vi "ecu_module.vi"(8 "error in (no error)":errorcluster, 10 "ecuData":refnum<user-event>, 11 "queue in":T1) -> (0 "error out":errorcluster)   [LabVIEW 2019]
uses:
  core_dataRef.ctl
  core_dataCluster.ctl
  gui/ecu_dataCluster.ctl
  instrument/Instrument.lvclass
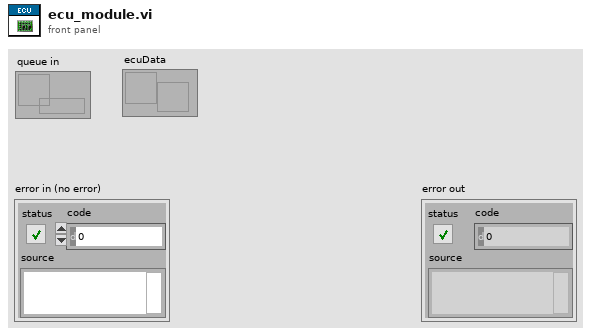
[diagram p1: front panel]
types:
  T1 = typedef "core_dataRef.ctl" = refnum<queue>
  T2 = typedef "ecu_dataCluster.ctl" = cluster{"MCU_MotCtrlrSts":dbl, "MCU_MotTq":dbl, "MCU_MotBusU":dbl, "MCU_MotSpd":dbl, "MCU_MotBodyT":dbl, "MCU_MotBody_T":dbl, "MCU_MotCtrlrT":dbl, "MCU 状态":bool, "ErrMsg":i64}
  T3 = typedef "core_dataCluster.ctl" = cluster{"cmd":string, "data":variant}
  T4 = typedef "Instrument.lvclass/DUT_Status.ctl" = cluster{"MCU_MotCtrlrSts":sgl, "MCU_MotTq":sgl, "MCU_MotBusU":sgl, "MCU_MotSpd":sgl}
  T5 = typedef "Instrument.lvclass/DUT_Temp.ctl" = cluster{"0x149_MCU_MotBodyT":sgl, "0x304_MCU_MotBodyT":sgl, "0x304_MCU_MotCtrlrT":sgl}
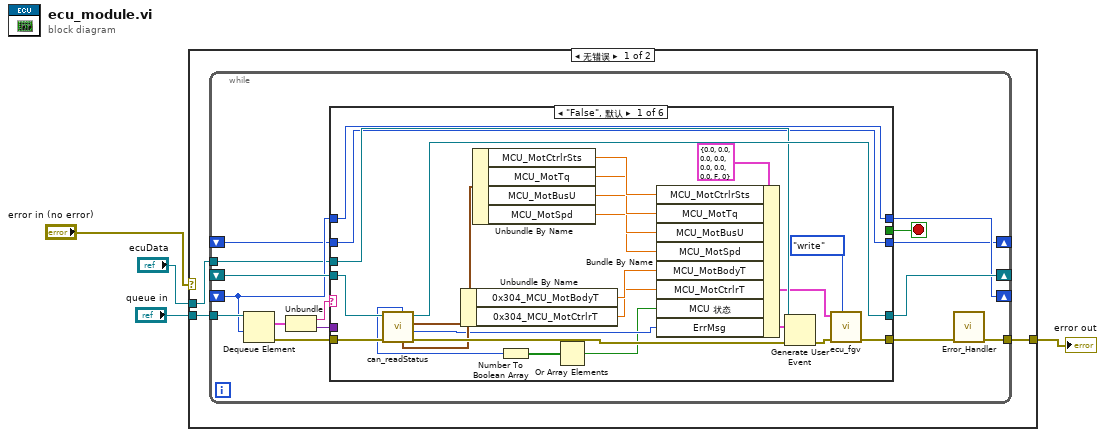
[diagram p0: block diagram]
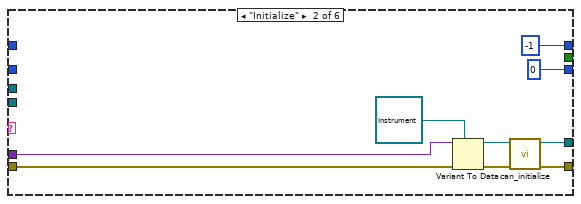
[diagram p2: hidden frame]
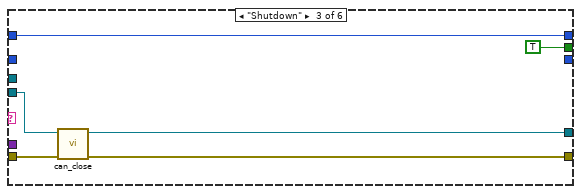
[diagram p3: hidden frame]
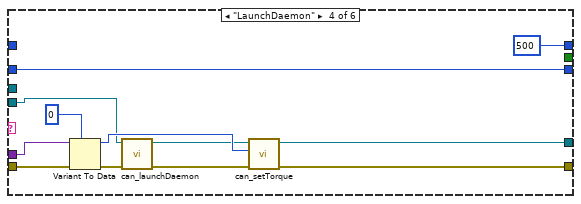
[diagram p4: hidden frame]
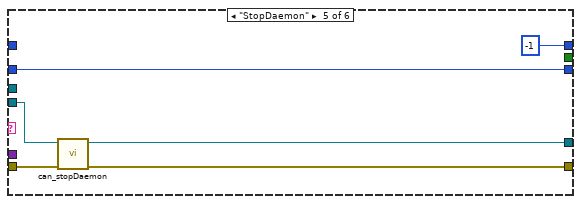
[diagram p5: hidden frame]
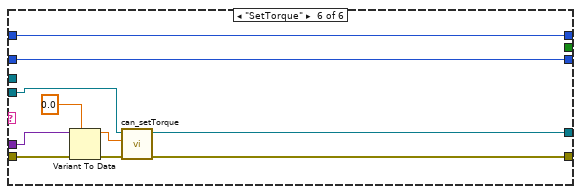
[diagram p6: hidden frame]
diagram:
  n1 = case shown="无错误" "error in (no error)" {
    selector: "error in (no error)" -> [_ w90]
    tunnel: "queue in" -> [w7 _]
    tunnel: [w6 w90] -> w3
    tunnel: "ecuData" -> [w5 _]
    frame No Error {
      n2 = while {
        tunnel: w7 -> [w22]
        shift-right: [w17] -> _
        shift-left: _ -> [w16]
        tunnel: [w14] -> w6
        shift-right: [w13] -> _
        shift-left: _ -> [w12]
        tunnel: w5 -> [w11]
        shift-right: [w10] -> _
        shift-left: _ -> [w9]
        stop <- w15 stop-if-true
        n3 = Dequeue Element(queue=w22, timeout in ms (-1)=w12) -> (element=w21:T3, error out=w19:errorcluster)  [unwired: 1 in, 2 out]
        n4 = Unbundle(w21) -> ("cmd"=w20:string, "data"=w18:variant)
        n5 = case shown="\"False\", 默认" w20 {
          tunnel: w19 -> [w43 w55 w57 w72 w78 w89]
          tunnel: w18 -> [_ w54 _ w71 _ w88]
          tunnel: [w44 w50 w61 w68 w77 w83] -> w17
          tunnel: w16 -> [w45 _ w58 w66 w79 w86]
          tunnel: [w39 w49 w60 w69 w76 w82] -> w8
          tunnel: [_ _ TRUE _ _ _] -> w15
          tunnel: [w46 -1 ("timeout in ms (-1)") w56 500 ("timeout in ms (-1)") -1 ("timeout in ms (-1)") w81] -> w13
          tunnel: w12 -> [w46 _ w56 _ _ w81]
          tunnel: w11 -> [w42 _ _ _ _ _]
          tunnel: [w37 u8 0 ("Control Mode") _ w64 w74 w80] -> w10
          tunnel: w9 -> [w37 _ _ w64 w74 w80]
          frame "False", Default {
            n6 = call "can_readStatus.vi"("error in (no error)"=w43, "Instrument in"=w45) -> ("error out"=w41:errorcluster, "FaultCode"=w26:u8, "Cluster"=w36:T4, "Instrument out"=w44:refnum<class "Instrument.lvclass">, "DUT_Temp"=w35:T5, "ReFltLvl"=w24:u8)  [unwired: 4 in]
            n7 = Unbundle By Name(w35) -> ("0x304_MCU_MotBodyT"=w28:sgl, "0x304_MCU_MotCtrlrT"=w27:sgl)
            n8 = Unbundle By Name(w36) -> ("MCU_MotCtrlrSts"=w32:sgl, "MCU_MotTq"=w31:sgl, "MCU_MotBusU"=w30:sgl, "MCU_MotSpd"=w29:sgl)
            n9 = Number To Boolean Array(number=w24) -> (Boolean array=w25:bool[])
            n10 = Or Array Elements(Boolean array=w25) -> (logical OR=w23:bool)
            n11 = Bundle By Name(cluster=T2 {"MCU_MotCtrlrSts"=0.0, "MCU_MotTq"=0.0, "MCU_MotBusU"=0.0, "MCU_MotSpd"=0.0, "MCU_MotBodyT"=0.0, "MCU_MotBody_T"=0.0, "MCU_MotCtrlrT"=0.0, "MCU 状态"=FALSE, "ErrMsg"=0} ("Cluster"), "MCU_MotCtrlrSts"=w32, "MCU_MotTq"=w31, "MCU_MotBusU"=w30, "MCU_MotSpd"=w29, "MCU_MotBodyT"=w28, "MCU_MotCtrlrT"=w27, "MCU 状态"=w23, "ErrMsg"=w26) -> (w33:T2)
            n12 = Generate User Event(user event=w42, event data cluster=w33, error in=w41) -> (error out=w40:errorcluster)  [unwired: 1 in, 1 out]
            n13 = call "ecu_fgv.vi"("mode"=enum16{"read", "write"}."write", "error in (no error)"=w40, "data in"=w33) -> ("error out"=w39:errorcluster)  [unwired: 7 in, 1 out]
          }
          frame "Initialize" {
            n14 = Variant To Data(error in=w55, type=refnum<class "Instrument.lvclass"> refnum ("Instrument.lvclass"), Variant=w54) -> (data=w51:refnum<class "Instrument.lvclass">, error out=w52:errorcluster)
            n15 = call "can_initialize.vi"("error in (no error)"=w52, "Instrument in"=w51) -> ("error out"=w49:errorcluster, "Instrument out"=w50:refnum<class "Instrument.lvclass">)  [unwired: 8 in]
          }
          frame "Shutdown" {
            n16 = call "can_close.vi"("error in (no error)"=w57, "Instrument in"=w58) -> ("error out"=w60:errorcluster, "Instrument out"=w61:refnum<class "Instrument.lvclass">)  [unwired: 8 in]
          }
          frame "LaunchDaemon" {
            n17 = Variant To Data(error in=w72, type=0, Variant=w71) -> (data=w70:i32, error out=w65:errorcluster)
            n18 = call "can_launchDaemon.vi"("error in (no error)"=w65, "Instrument in"=w66) -> ("error out"=w63:errorcluster, "Instrument out"=w62:refnum<class "Instrument.lvclass">)  [unwired: 8 in]
            n19 = call "can_setTorque.vi"("error in (no error)"=w63, "Torque"=w70, "Instrument in"=w62) -> ("error out"=w69:errorcluster, "Instrument out"=w68:refnum<class "Instrument.lvclass">)  [unwired: 7 in]
          }
          frame "StopDaemon" {
            n20 = call "can_stopDaemon.vi"("error in (no error)"=w78, "Instrument in"=w79) -> ("error out"=w76:errorcluster, "Instrument out"=w77:refnum<class "Instrument.lvclass">)  [unwired: 8 in]
          }
          frame "SetTorque" {
            n21 = Variant To Data(error in=w89, type=sgl 0.0, Variant=w88) -> (data=w85:sgl, error out=w84:errorcluster)
            n22 = call "can_setTorque.vi"("error in (no error)"=w84, "Torque"=w85, "Instrument in"=w86) -> ("error out"=w82:errorcluster, "Instrument out"=w83:refnum<class "Instrument.lvclass">)  [unwired: 7 in]
          }
        }
        n23 = call "Error_Handler.vi"("error in"=w8) -> ("error out"=w14:errorcluster)  [unwired: 8 in, 2 out]
      }
    }
    frame Error {
    }
  }
  "error out" <- w3
